vi "Agilent VNA Set Power.vi"(6 "Channel":i8=1 min=1 max=99 step=1, 7 "Agilent VNA":T1, 8 "error in (no error)":errorcluster, 10 "Source Power, dBm (0.0)":dbl, 11 "VISA Resource Name":refnum<visa-resource-name>) -> (0 "error out":errorcluster, 3 "dup VISA Resource Name":refnum<visa-resource-name>)   [LabVIEW 2011]
doc: "This vi sets the power range. Only works on the HP 8753D."
uses:
  TypeDefs/Agilent VNA Instrument Info.ctl
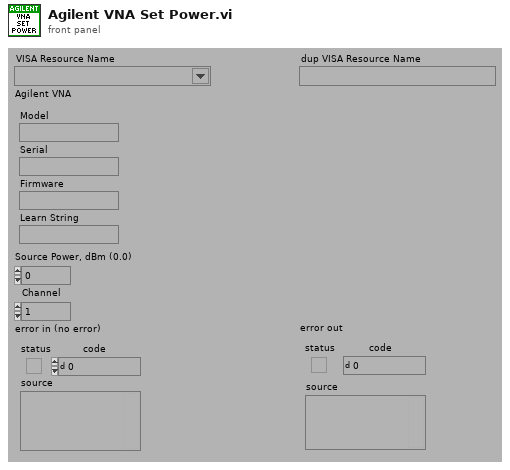
[diagram p1: front panel]
types:
  T1 = typedef "Agilent VNA Instrument Info.ctl" = cluster{"Model":string, "Serial":string, "Firmware":string, "Learn String":string}
  T2 = typedef "Agilent VNA Model.ctl" = enum16{"Not Supported", "8510X", "8719X", "8720X", "8722X", "8753X", "ENA", "PNA", "Field Fox"}
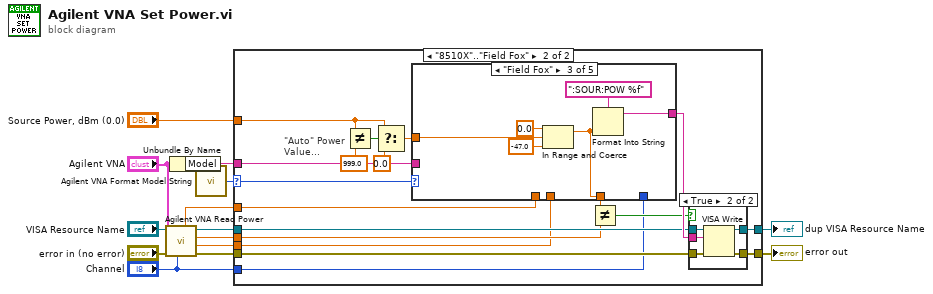
[diagram p0: block diagram]
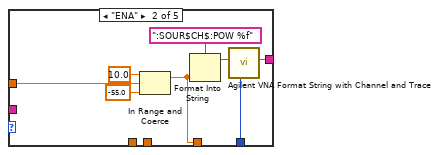
[diagram p4: hidden frame]
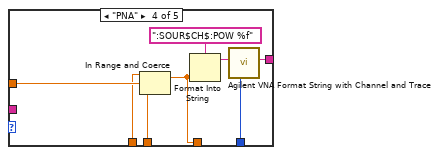
[diagram p5: hidden frame]
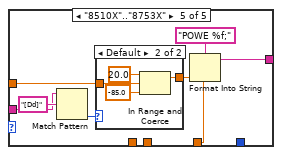
[diagram p6: hidden frame]
diagram:
  n1 = call "Agilent VNA Read Power.vi"("Channel"="Channel", "Agilent VNA"="Agilent VNA", "error in (no error)"="error in (no error)", "VISA Resource Name"="VISA Resource Name") -> ("error out"=w11:errorcluster, "Source Power Min, dBm"=w6:dbl, "Source Power, dBm"=w8:dbl, "dup VISA Resource Name"=w9:refnum<visa-resource-name>, "Source Power Max, dBm"=w5:dbl)  [unwired: 3 out]
  n2 = Unbundle By Name("Agilent VNA") -> ("Model"=w1:string)
  n3 = call "Agilent VNA Format Model String.vi"("Model"=w1) -> ("Model"=w2:T2)
  n4 = case shown="\"8510X\"..\"Field Fox\"" w2 {
    selector: w2 -> [_ w18]
    tunnel: [w15 w34] -> w14
    tunnel: [w16 w33] -> w13
    tunnel: w11 -> [w15 w30]
    tunnel: w9 -> [w16 w29]
    tunnel: w8 -> [_ w28]
    tunnel: "Source Power, dBm (0.0)" -> [_ w23]
    tunnel: w6 -> [_ w21]
    tunnel: w5 -> [_ w20]
    tunnel: "Channel" -> [_ w19]
    tunnel: w1 -> [_ w17]
    frame "Not Supported" {
    }
    frame "8510X".."Field Fox" {
      # "\"Auto\" Power\nValue..."
      n5 = Not Equal?(x=w23, y=999.0) -> (x != y?=w24:bool)
      n6 = Select(t=w23, s=w24, f=0.0) -> (s? t:f=w22:dbl)
      n7 = case shown="\"Field Fox\"" w18 {
        tunnel: [_ w36 w43 w52 w62] -> w31
        tunnel: w22 -> [_ w39 w45 w55 w60]
        tunnel: [_ w38 w44 w54 w61] -> w26
        tunnel: w21 -> [_ _ _ w51 _]
        tunnel: w20 -> [_ _ _ w50 _]
        tunnel: w19 -> [_ w35 _ w49 _]
        tunnel: w17 -> [_ _ _ _ w57]
        frame "Not Supported" {
        }
        frame "ENA" {
          n8 = In Range and Coerce(upper limit=10.0, x=w39, lower limit=-55.0) -> (coerced(x)=w38:dbl)  [unwired: 1 out]
          n9 = Format Into String(format string=":SOUR$CH$:POW %f", w38) -> (resulting string=w37:string)  [unwired: 2 in, 1 out]
          n10 = call "Agilent VNA Format String with Channel and Trace.vi"("Channel"=w35, "String"=w37) -> ("String Out"=w36:string)  [unwired: 1 in, 6 out]
        }
        frame "Field Fox" {
          n11 = In Range and Coerce(upper limit=0.0, x=w45, lower limit=-47.0) -> (coerced(x)=w44:dbl)  [unwired: 1 out]
          n12 = Format Into String(format string=":SOUR:POW %f", w44) -> (resulting string=w43:string)  [unwired: 2 in, 1 out]
        }
        frame "PNA" {
          n13 = In Range and Coerce(upper limit=w50, x=w55, lower limit=w51) -> (coerced(x)=w54:dbl)  [unwired: 1 out]
          n14 = Format Into String(format string=":SOUR$CH$:POW %f", w54) -> (resulting string=w53:string)  [unwired: 2 in, 1 out]
          n15 = call "Agilent VNA Format String with Channel and Trace.vi"("Channel"=w49, "String"=w53) -> ("String Out"=w52:string)  [unwired: 1 in, 6 out]
        }
        frame "8510X".."8753X" {
          n16 = Match Pattern(string=w57, regular expression="[Dd]") -> (offset past match=w58:i32)  [unwired: 4 out]
          n17 = case shown="Default" w58 {
            tunnel: w60 -> [w64 w68]
            tunnel: [w64 w65] -> w61
            frame -1 {
            }
            frame Default {
              n18 = In Range and Coerce(upper limit=20.0, x=w68, lower limit=-85.0) -> (coerced(x)=w65:dbl)  [unwired: 1 out]
            }
          }
          n19 = Format Into String(format string="POWE %f;", w61) -> (resulting string=w62:string)  [unwired: 2 in, 1 out]
        }
      }
      n20 = Not Equal?(x=w26, y=w28) -> (x != y?=w27:bool)
      n21 = case shown="True" w27 {
        tunnel: [w69 w75] -> w34
        tunnel: [w70 w74] -> w33
        tunnel: w31 -> [_ w73]
        tunnel: w30 -> [w69 w72]
        tunnel: w29 -> [w70 w71]
        frame False {
        }
        frame True {
          n22 = VISA Write(VISA resource name=w71, write buffer=w73, error in (no error)=w72) -> (VISA resource name out=w74:refnum<visa-resource-name>, error out=w75:errorcluster)  [unwired: 1 out]
        }
      }
    }
  }
  "dup VISA Resource Name" <- w13
  "error out" <- w14
